vi "sub_check-ip.vi"() -> (2 "ip output":string, 3 "standard output":string)   [LabVIEW 2019]
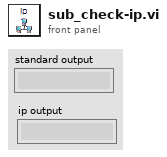
[diagram p1: front panel]
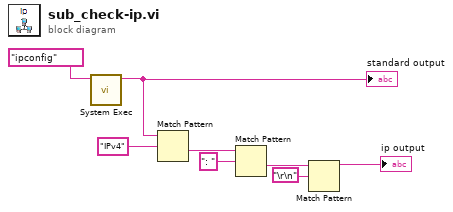
[diagram p0: block diagram]
diagram:
  n1 = call <vilib>:"System Exec.vi"("command line"="ipconfig") -> ("standard output"=w7:string)  [unwired: 7 in, 3 out]
  "standard output" <- w7
  n2 = Match Pattern(string=w7, regular expression="IPv4" ("정규식")) -> (after substring=w4:string)  [unwired: 1 in, 3 out]
  n3 = Match Pattern(string=w4, regular expression=": " ("정규식")) -> (after substring=w6:string)  [unwired: 1 in, 3 out]
  n4 = Match Pattern(string=w6, regular expression="\r\n") -> (before substring=→"ip output":string)  [unwired: 1 in, 3 out]
